vi "Schedule.vi"(2 "error in (no error)":errorcluster, 3 "Schedule":cluster{"UTC ON hour":i32, "UTC OFF hour":i32}={"UTC ON hour"=22, "UTC OFF hour"=8}) -> (0 "error out":errorcluster, 1 "True: record":bool)   [LabVIEW 2014]
doc: "Enables recording during sunset (unless ALLSTOP = True)"
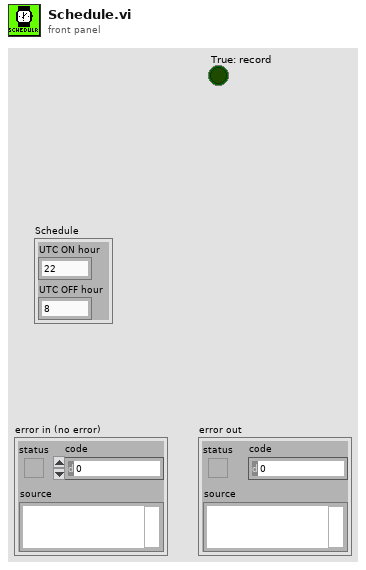
[diagram p1: front panel]
types:
  T1 = typedef "LVDateTimeRec.ctl" = cluster{"fractional second":dbl, "second":i32, "minute":i32, "hour":i32, "day of month":i32, "month":i32, "year":i32, "day of week":i32, "day of year":i32, "DST":i32}
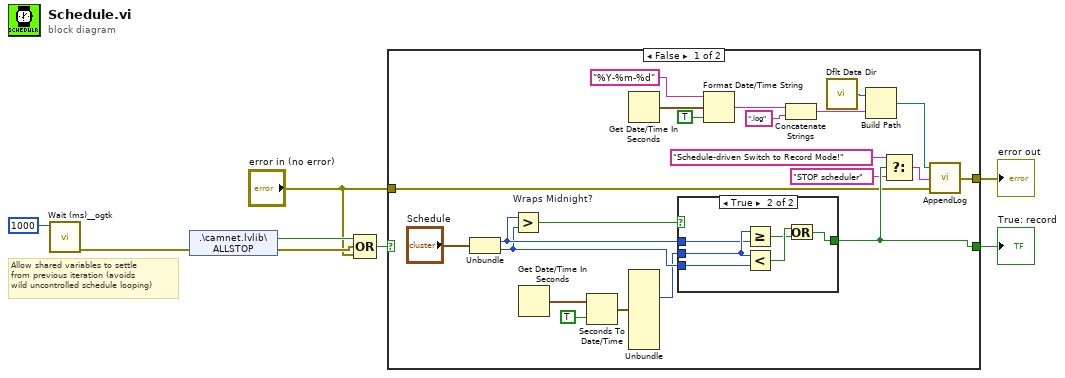
[diagram p0: block diagram]
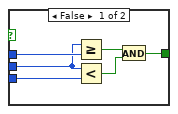
[diagram p2: hidden frame]
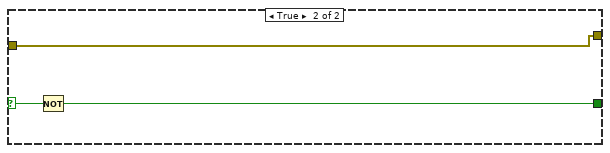
[diagram p3: hidden frame]
diagram:
  # "Allow shared variables to settle\nfrom previous iteration (avoids\nwild uncontrolled schedule looping)"
  n1 = call <userlib>:"Wait (ms)__ogtk.vi"("milliseconds to wait"=u32 1000) -> ("error out"=w3:errorcluster)  [unwired: 9 in, 1 out]
  n2 = shared-variable ".\\camnet.lvlib\\ALLSTOP"(error in=w3) -> (w7:bool, error out=w8:errorcluster)
  n3 = Compound Arithmetic op=OR(w7, w8, "error in (no error)") -> (w6:bool)
  n4 = case shown="False" w6 {
    selector: w6 -> [_ w44]
    tunnel: [w17 w45] -> w4
    tunnel: [w19 w43] -> w5
    tunnel: "error in (no error)" -> [w9 w45]
    frame False {
      n5 = Unbundle("Schedule") -> ("UTC ON hour"=w22:i32, "UTC OFF hour"=w21:i32)
      n6 = Greater? "Wraps Midnight?"(x=w22, y=w21) -> (0:w10:bool)
      n7 = Get Date/Time In Seconds() -> (seconds since 1Jan1904=w12:timestamp)
      n8 = Seconds To Date/Time(time stamp (now)=w12, to UTC (F)=TRUE) -> (date time rec=w14:T1)
      n9 = Get Date/Time In Seconds() -> (seconds since 1Jan1904=w27:timestamp)
      n10 = Unbundle(w14) -> ("hour"=w11:i32)  [unwired: 9 out]
      n11 = case shown="True" w10 {
        tunnel: w11 -> [w34 w41]
        tunnel: [w31 w39] -> w19
        tunnel: w22 -> [w36 w38]
        tunnel: w21 -> [w35 w37]
        frame False {
          n12 = Greater Or Equal?(x=w34, y=w36) -> (x >= y?=w33:bool)
          n13 = Less?(x=w34, y=w35) -> (x < y?=w32:bool)
          n14 = And(x=w33, y=w32) -> (x .and. y?=w31:bool)
        }
        frame True {
          n15 = Greater Or Equal?(x=w41, y=w38) -> (x >= y?=w40:bool)
          n16 = Less?(x=w41, y=w37) -> (x < y?=w42:bool)
          n17 = Or(x=w42, y=w40) -> (x .or. y?=w39:bool)
        }
      }
      n18 = Format Date/Time String(time format string (%c)="%Y-%m-%d", seconds (now)=w27, UTC format=TRUE) -> (date/time string=w24:string)
      n19 = Concatenate Strings(w24, ".log" ("string")) -> (w28:string)
      n20 = call <vilib>:"Dflt Data Dir.vi"() -> ("App:Default Data Directory"=w29:path)
      n21 = Build Path(base path=w29, name or relative path=w28) -> (appended path=w20:path)
      n22 = Select(t="Schedule-driven Switch to Record Mode!" ("String"), s=w19, f="STOP scheduler" ("t")) -> (s? t:f=w18:string)
      n23 = call "AppendLog.vi"("error in"=w9, "text to write"=w18, "file path (use dialog)"=w20) -> ("error out"=w17:errorcluster)
    }
    frame True {
      n24 = Not(x=w44) -> (.not. x?=w43:bool)
    }
  }
  "True: record" <- w5
  "error out" <- w4
